vi "Queue-Driven State Machine Example.vi"() -> ()   [LabVIEW 2018]
uses:
  <vilib>/Utility/error.llb/Error Cluster From Error Code.vi
  <vilib>/ErrorRing/Error Ring.xnode
panel:
  in  "Stop":bool
  in  "Test 2":bool
  in  "Test 1":bool
  # "Event-Drivend Queued State Machine"
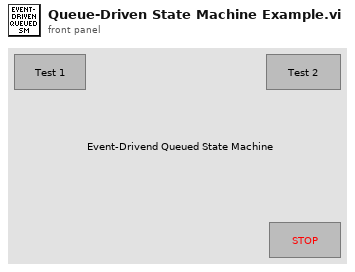
[diagram p1: front panel]
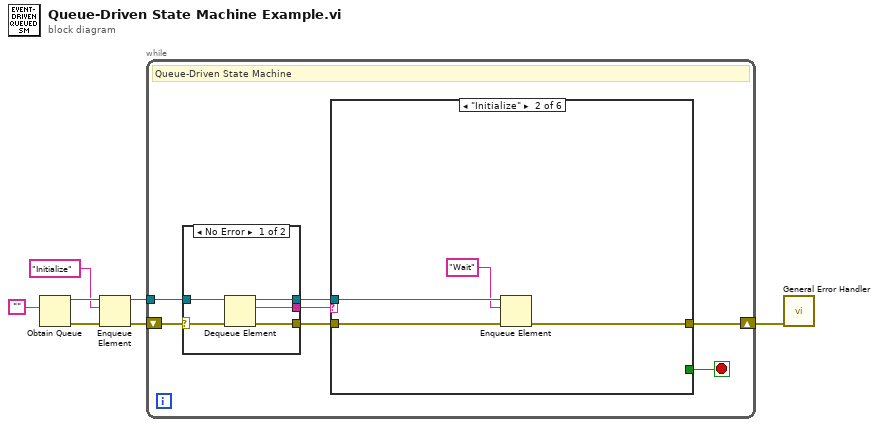
[diagram p0: block diagram]
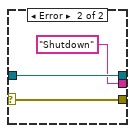
[diagram p2: hidden frame]
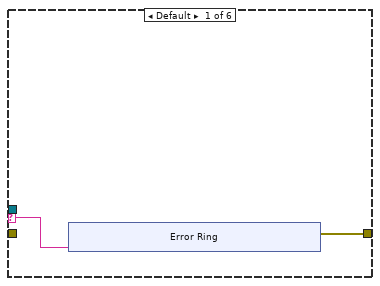
[diagram p3: hidden frame]
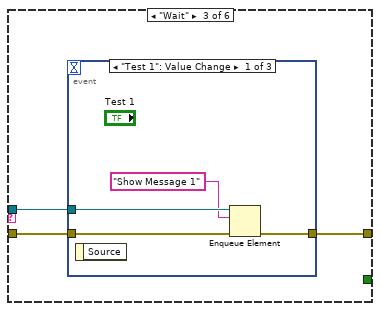
[diagram p4: hidden frame]
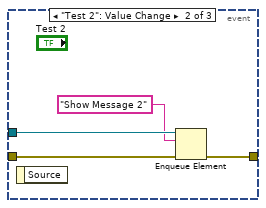
[diagram p5: hidden frame]
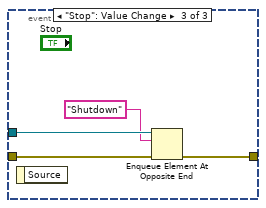
[diagram p6: hidden frame]
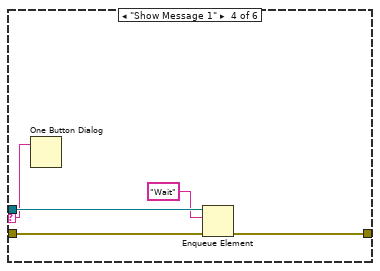
[diagram p7: hidden frame]
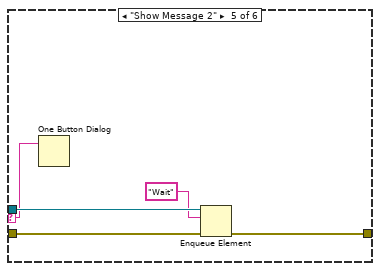
[diagram p8: hidden frame]
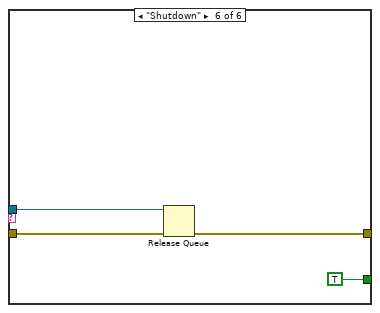
[diagram p9: hidden frame]
diagram:
  n1 = Obtain Queue(element data type="" ("name (unnamed)")) -> (queue out=w5:refnum<queue>, error out=w6:errorcluster)  [unwired: 4 in, 1 out]
  n2 = Enqueue Element(queue=w5, element="Initialize", error in (no error)=w6) -> (queue out=w4:refnum<queue>, error out=w3:errorcluster)  [unwired: 1 in, 1 out]
  n3 = while {
    tunnel: w4 -> [w14]
    shift-right: [w10] -> w1
    shift-left: w3 -> [w8]
    stop <- w9 stop-if-true
    # "Queue-Driven State Machine"
    n4 = case shown="No Error" w8 {
      selector: w8 -> [w15 w20]
      tunnel: w14 -> [w19 w22]
      tunnel: [w18 w20] -> w13
      tunnel: [w17 w22] -> w12
      tunnel: [w16 "Shutdown"] -> w11
      frame No Error {
        n5 = Dequeue Element(queue=w19, error in (no error)=w15) -> (queue out=w17:refnum<queue>, element=w16:string, error out=w18:errorcluster)  [unwired: 1 in, 1 out]
      }
      frame Error {
      }
    }
    n6 = case shown="\"Initialize\"" w11 {
      selector: w11 -> [w23 _ _ w54 w59 _]
      tunnel: w13 -> [_ w35 w38 w53 w58 w64]
      tunnel: w12 -> [_ w33 w37 w55 w60 w62]
      tunnel: [w24 w34 w36 w52 w57 w63] -> w10
      tunnel: [_ _ _ _ _ TRUE] -> w9
      frame Default {
        n7 = xnode "Error Ring"("parameter 0"=w23) -> ("error out"=w24:errorcluster)
      }
      frame "Initialize" {
        n8 = Enqueue Element(queue=w33, element="Wait", error in (no error)=w35) -> (error out=w34:errorcluster)  [unwired: 1 in, 2 out]
      }
      frame "Wait" {
        n9 = event shown="[0] \"Test 1\": Value Change" {
          selector: _ -> [_ _ _]
          dyn-events: _ -> [_ _ _]
          timeout: _ -> [_ _ _]
          tunnel: w38 -> [w42 w44 w50]
          tunnel: w37 -> [w40 w46 w48]
          tunnel: [w41 w43 w49] -> w36
          event "Test 1": Value Change {
            n10 = event-data() -> ()  [unwired: 1 in, 1 out]
            n11 = Enqueue Element(queue=w40, element="Show Message 1", error in (no error)=w42) -> (error out=w41:errorcluster)  [unwired: 1 in, 2 out]
          }
          event "Test 2": Value Change {
            n12 = event-data() -> ()  [unwired: 1 in, 1 out]
            n13 = Enqueue Element(queue=w46, element="Show Message 2", error in (no error)=w44) -> (error out=w43:errorcluster)  [unwired: 1 in, 2 out]
          }
          event "Stop": Value Change {
            n14 = event-data() -> ()  [unwired: 1 in, 1 out]
            n15 = Enqueue Element At Opposite End(queue=w48, element="Shutdown", error in (no error)=w50) -> (error out=w49:errorcluster)  [unwired: 1 in, 2 out]
          }
        }
      }
      frame "Show Message 1" {
        n16 = One Button Dialog(message=w54) -> ()  [unwired: 1 in, 1 out]
        n17 = Enqueue Element(queue=w55, element="Wait", error in (no error)=w53) -> (error out=w52:errorcluster)  [unwired: 1 in, 2 out]
      }
      frame "Show Message 2" {
        n18 = One Button Dialog(message=w59) -> ()  [unwired: 1 in, 1 out]
        n19 = Enqueue Element(queue=w60, element="Wait", error in (no error)=w58) -> (error out=w57:errorcluster)  [unwired: 1 in, 2 out]
      }
      frame "Shutdown" {
        n20 = Release Queue(queue=w62, error in (no error)=w64) -> (error out=w63:errorcluster)  [unwired: 1 in, 2 out]
      }
    }
  }
  n21 = call <vilib>:"General Error Handler.vi"("error in (no error)"=w1) -> ()  [unwired: 10 in, 5 out]
